vi "Draw Scalable Border.vi"(8 "error in (no error)":errorcluster, 9 "Bounds":cluster{"Width":u32, "Height":u32}, 10 "Position":cluster{"Left":i32, "Top":i32}, 11 "2 Points Border in":refnum<class "2 Points Border.lvclass">) -> (0 "error out":errorcluster, 2 "Border out":picture, 3 "2 Points Border out":refnum<class "2 Points Border.lvclass">)   [LabVIEW 2015, in "2 Points Border.lvclass"]
uses:
  2 Points Border.lvclass
panel:
  # "NOTICE -- YOU MUST LEAVE THIS NOTICE IN PLACE.\n\nCopyright (c) 2017, LIANG LIU Shawn.Liu.cn@gmail.com\nAll rights reserved.\n\nRedistribution and use in source and binary forms, with or without modification, are permitted provided that the following conditions are met:\n-Redistributions of source code must retain the above copyright notice, this list of conditions and the following disclaimer.\n-Redistributions in binary form must reproduce the above copyright notice, this list of conditions and the following disclaimer in the documentation and/or other materials provided with the distribution.\n-Neither the name of the eLp nor the names of its contributors may be used to endorse or promote products derived from this software without specific prior written permission.\n\nTHIS SOFTWARE IS PROVIDED BY THE COPYRIGHT HOLDERS AND CONTRIBUTORS \"AS IS\" AND ANY EXPRESS OR IMPLIED WARRANTIES, INCLUDING, BUT NOT LIMITED TO, THE IMPLIED WARRANTIES OF MERCHANTABILITY AND FITNESS FOR A PARTICULAR PURPOSE ARE DISCLAIMED. IN NO EVENT SHALL THE COPYRIGHT HOLDER OR CONTRIBUTORS BE LIABLE FOR ANY DIRECT, INDIRECT, INCIDENTAL, SPECIAL, EXEMPLARY, OR CONSEQUENTIAL DAMAGES (INCLUDING, BUT NOT LIMITED TO, PROCUREMENT OF SUBSTITUTE GOODS OR SERVICES; LOSS OF USE, DATA, OR PROFITS; OR BUSINESS INTERRUPTION) HOWEVER CAUSED AND ON ANY THEORY OF LIABILITY, WHETHER IN CONTRACT, STRICT LIABILITY, OR TORT (INCLUDING NEGLIGENCE OR OTHERWISE) ARISING IN ANY WAY OUT OF THE USE OF THIS SOFTWARE, EVEN IF ADVISED OF THE POSSIBILITY OF SUCH DAMAGE."
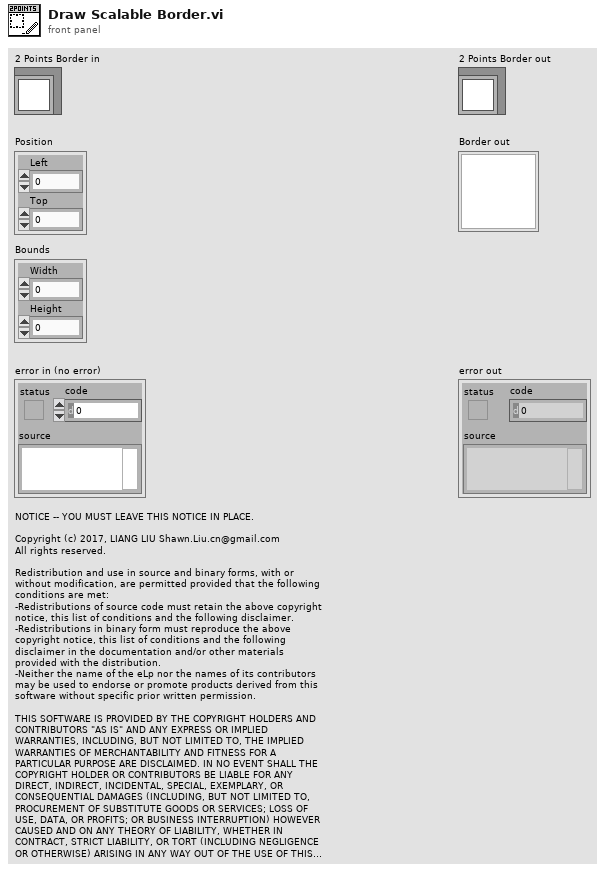
[diagram p1: front panel]
types:
  T1 = cluster{"left":i16, "top":i16, "right":i16, "bottom":i16}
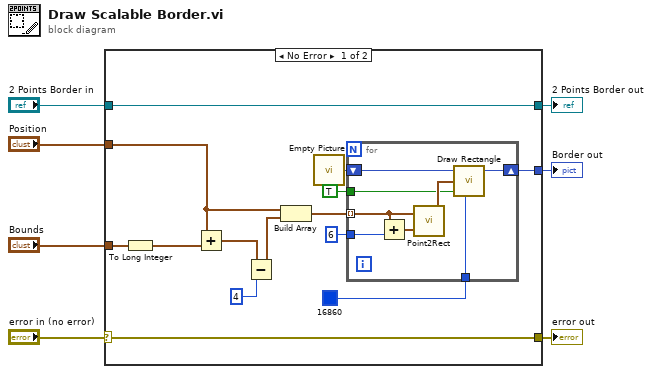
[diagram p0: block diagram]
diagram:
  n1 = case shown="No Error" "error in (no error)" {
    selector: "error in (no error)" -> [w10 w31]
    tunnel: "Bounds" -> [w12 _]
    tunnel: "Position" -> [w11 _]
    tunnel: [w10 w31] -> w4
    tunnel: [w9 _] -> w3
    tunnel: "2 Points Border in" -> [w8 w30]
    tunnel: [w8 w30] -> w1
    frame No Error {
      n2 = To Long Integer(number=w12) -> (32bit integer=w21:cluster{"Width":i32, "Height":i32})
      n3 = Add(x=w11, y=w21) -> (x+y=w13:cluster{i32, i32})
      n4 = Subtract(x=w13, y=4) -> (x-y=w19:cluster{i32, i32})
      n5 = Build Array(w11, w19) -> (w18:cluster{"Left":i32, "Top":i32}[])
      n6 = call "Empty Picture"() -> ("empty picture"=w17:picture)
      n7 = for {
        tunnel: w18 -> [w28] mode=indexing
        shift-right: [w25] -> w9
        shift-left: w17 -> [w29]
        tunnel: TRUE -> [w24]
        tunnel: 6 -> [w23]
        tunnel: u32 16860 -> [w22]
        n8 = Add(x=w28, y=w23) -> (x+y=w27:cluster{"Left":i32, "Top":i32})
        n9 = call <vilib>:"Point2Rect.vi"("point b"=w27, "point a"=w28) -> ("rect"=w26:T1)
        n10 = call <vilib>:"Draw Rectangle.vi"("picture"=w29, "rect"=w26, "fill?(F)"=w24, "color(black)"=w22) -> ("new picture"=w25:picture)  [unwired: 5 in]
      }
    }
    frame Error {
    }
  }
  "error out" <- w4
  "2 Points Border out" <- w1
  "Border out" <- w3
